vi "InstrumentStudio Plug-In Template.vi"() -> ()   [LabVIEW 2021, in "InstrumentStudio Plug-In Template.lvlib"]
uses:
  InstrumentStudio Plug-In Template.lvlib
  <vilib>/Plug-In SDKs/InstrumentStudio/Plugin Events Enum.ctl
  <vilib>/Plug-In SDKs/InstrumentStudio/Plugin Session.lvclass
  <vilib>/Plug-In SDKs/InstrumentStudio/InstrumentStudio Plugin SDK.lvlib
panel:
  in  "Tab Control":T1(tab)
  in  "Read Selected Sites":bool
  in  "Read Active Pin Map Path":bool
  out "Sites":i32[](array[numeric])
  out "Project Path":path
  in  "Run Write":string
  in  "Write Run Time Config":bool
  in  "Edit Write":string
  in  "Write Edit Time Config":bool
  out "Run Read":string
  in  "Read Run Time Config":bool
  out "Edit Read":string
  in  "Read Edit Time Config":bool
  in  "Read Project Path":bool
  in  "Running":bool
  out "Active Pin Map Path":path
  out "Event Record":i32(listbox)
  in  "Session Id":u64
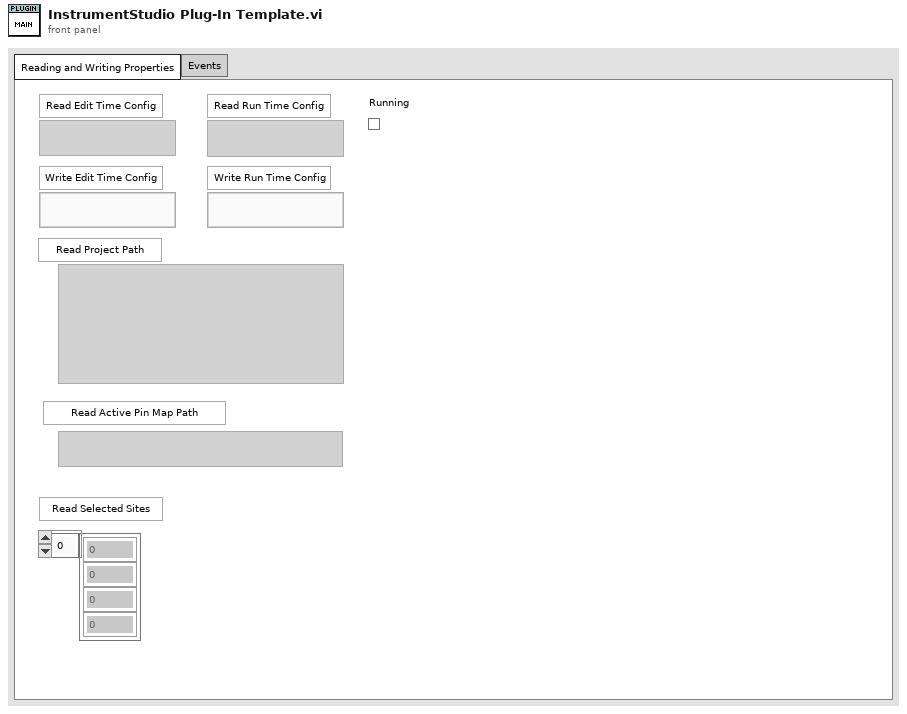
[diagram p1: front panel]
types:
  T1 = enum32{"Reading and Writing Properties", "Events"}
  T2 = typedef "InstrumentStudio Plugin SDK.lvlib/Plugin Events Enum.ctl" = enum32{"Shutdown", "Project Saved", "Stop All Outputs", "Generic Message", "Active Pin Map Changed", "Selected Sites Changed"}
  T3 = typedef "InstrumentStudio Plugin SDK.lvlib/Event Registration Refnum.ctl" = refnum<event-registration>
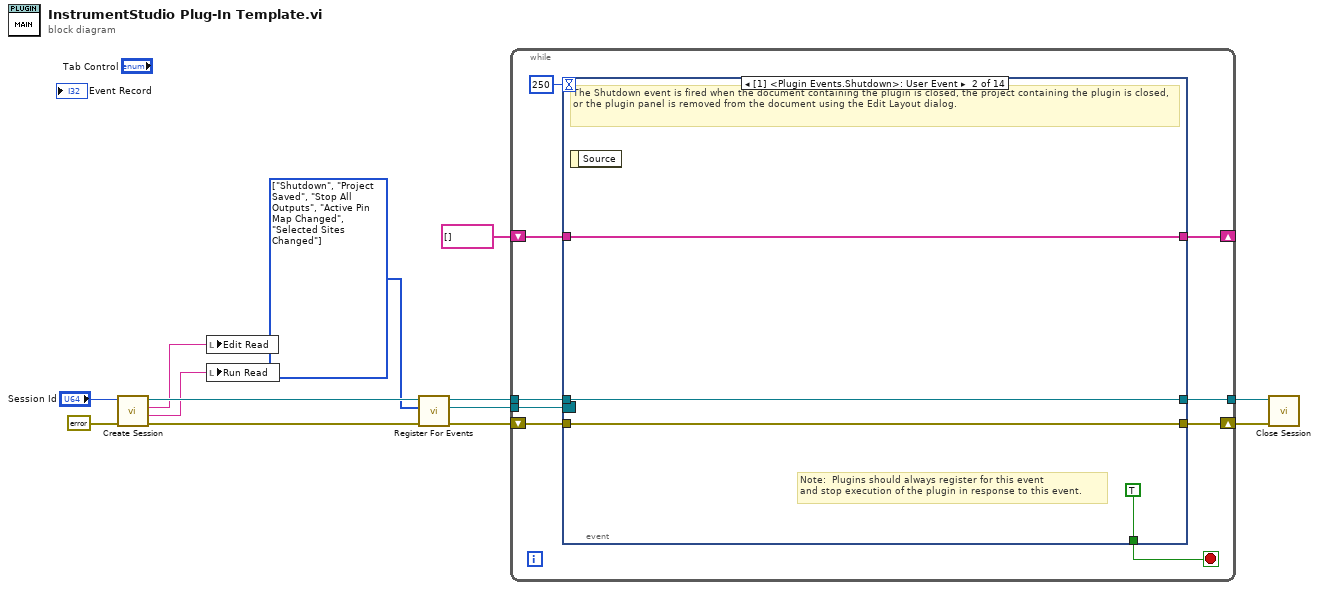
[diagram p0: block diagram]
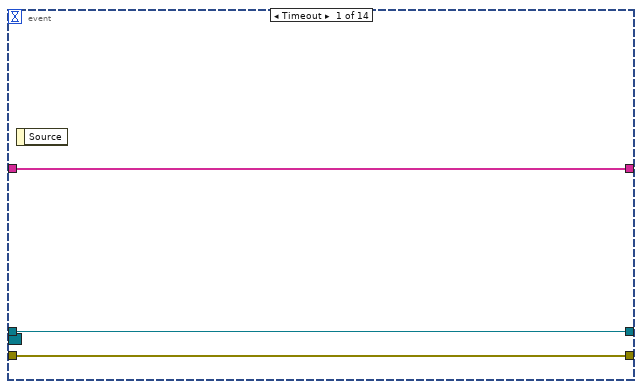
[diagram p2: hidden frame]
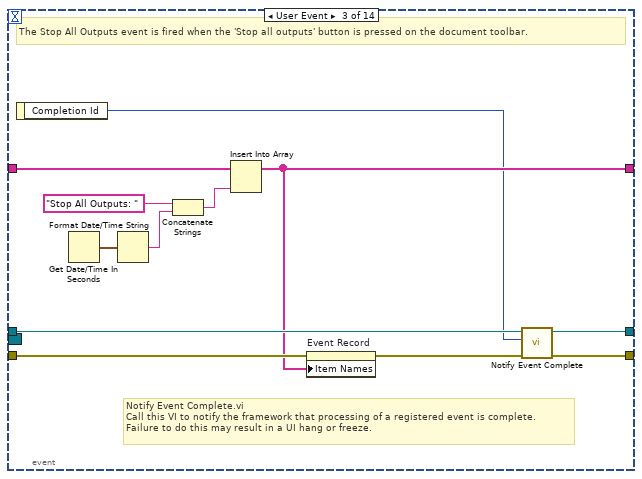
[diagram p3: hidden frame]
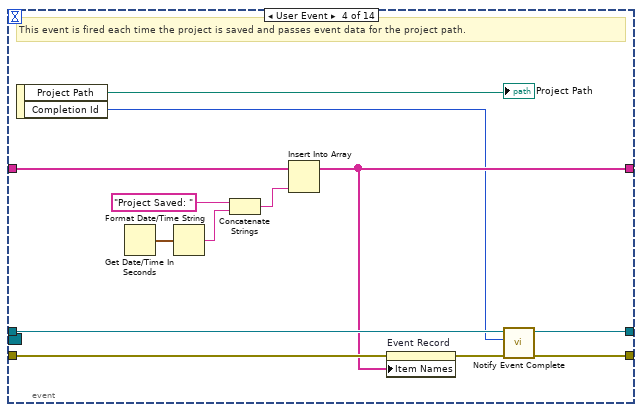
[diagram p4: hidden frame]
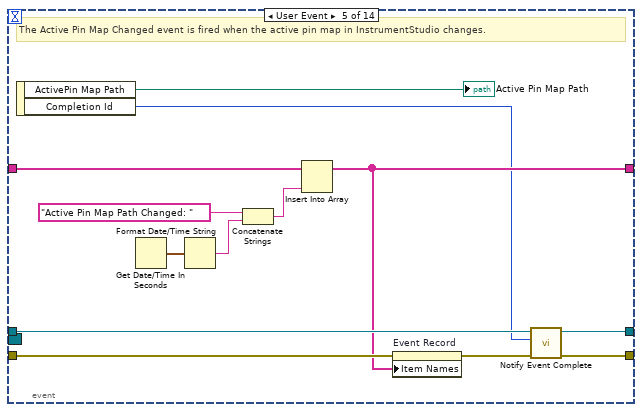
[diagram p5: hidden frame]
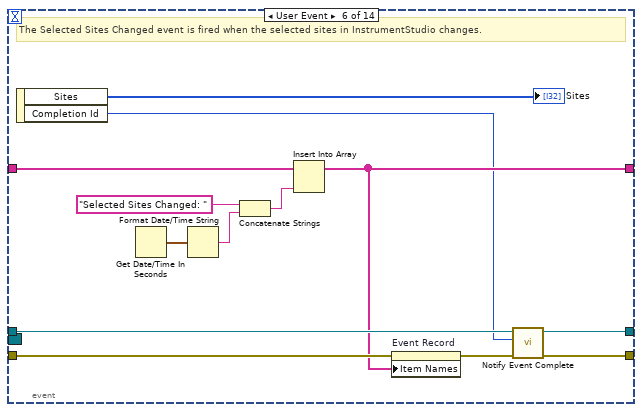
[diagram p6: hidden frame]
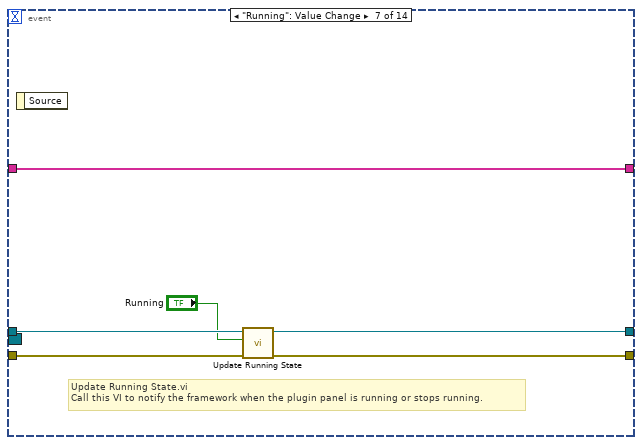
[diagram p7: hidden frame]
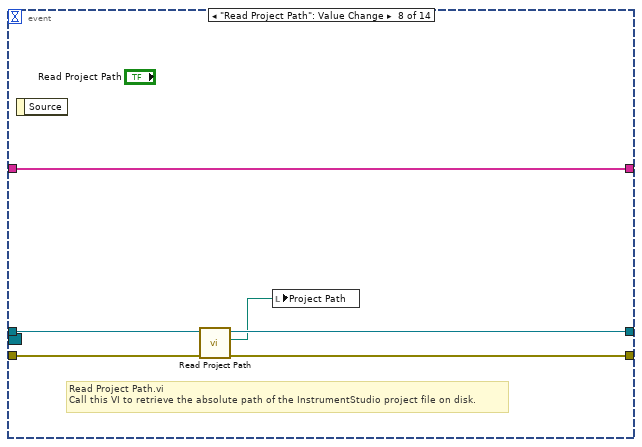
[diagram p8: hidden frame]
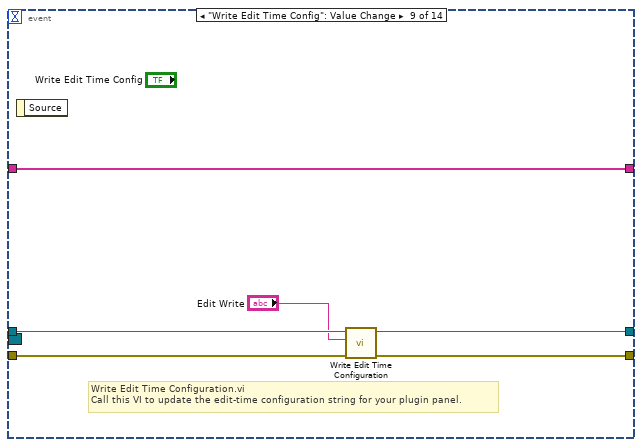
[diagram p9: hidden frame]
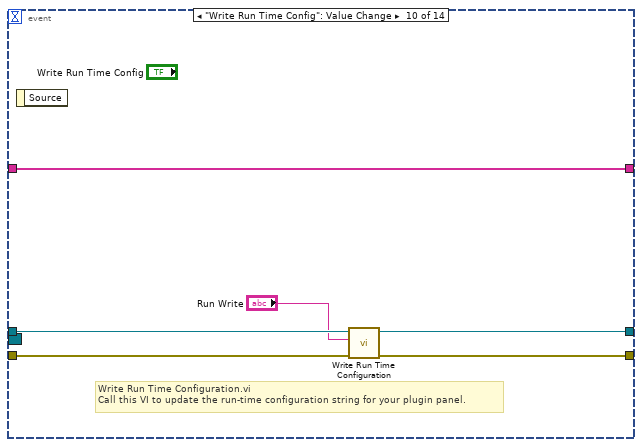
[diagram p10: hidden frame]
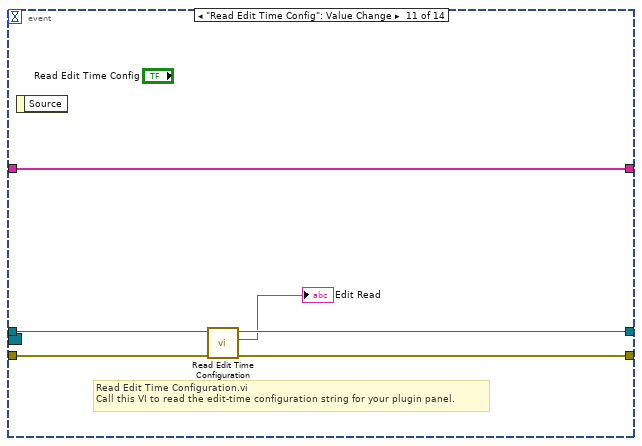
[diagram p11: hidden frame]
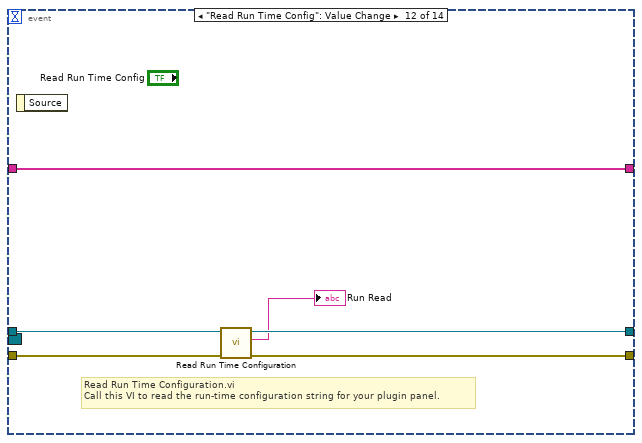
[diagram p12: hidden frame]
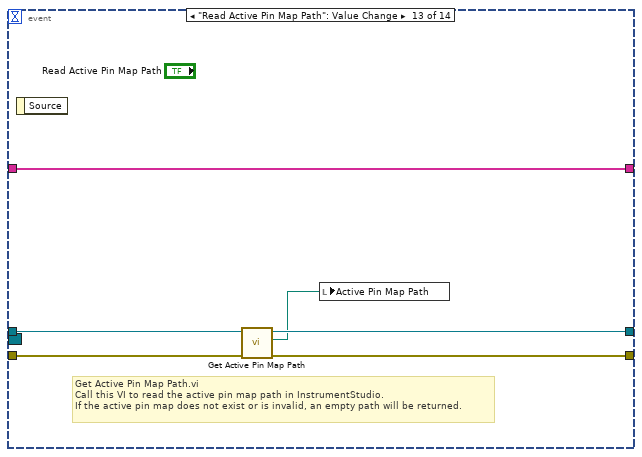
[diagram p13: hidden frame]
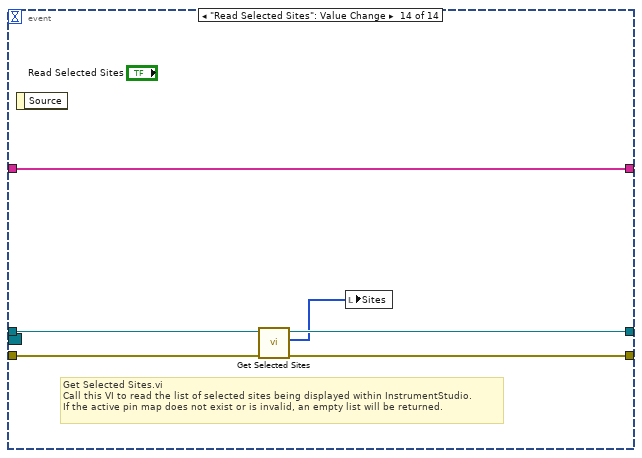
[diagram p14: hidden frame]
diagram:
  w3 = T2[] [enum."Shutdown", enum."Project Saved", enum."Stop All Outputs", enum."Active Pin Map Changed", enum."Selected Sites Changed"] items=["Shutdown", "Project Saved", "Stop All Outputs", "Generic Message", "Active Pin Map Changed", "Selected Sites Changed"] ("Events To Register")
  n1 = call <vilib>:"Create Session.vi"("error in (no error)"=errorcluster {"status"=FALSE, "code"=0, "source"=""}, "Session Id"="Session Id") -> ("error out"=w10:errorcluster, "Run Time Configuration"=w6:string, "Edit Time Configuration"=w5:string, "Session out"=w12:refnum<class "Plugin Session.lvclass">)  [unwired: 5 in, 1 out]
  n2 = local write "Edit Read"(w5) -> ()
  n3 = local write "Run Read"(w6) -> ()
  n4 = call <vilib>:"Register For Events.vi"("error in (no error)"=w10, "Events To Register"=w3, "Session in"=w12) -> ("error out"=w8:errorcluster, "Event Refnum"=w9:T3, "Session out"=w11:refnum<class "Plugin Session.lvclass">)  [unwired: 6 in]
  n5 = while {
    tunnel: w11 -> [w22]
    tunnel: w9 -> [w16]
    shift-right: [w21] -> w1
    shift-left: w8 -> [w18]
    shift-right: [w20] -> _
    shift-left: string[] [] -> [w19]
    tunnel: [w15] -> w2
    stop <- w17 stop-if-true
    n6 = event shown="[1] <Plugin Events.Shutdown>: User Event" {
      selector: w16 -> [_ _ _ _ _ _ _ _ _ _ _ _ _ _]
      dyn-events: _ -> [_ _ _ _ _ _ _ _ _ _ _ _ _ _]
      timeout: 250 -> [_ _ _ _ _ _ _ _ _ _ _ _ _ _]
      tunnel: w22 -> [w25 w29 w41 w54 w67 w79 w86 w92 w97 w100 w106 w112 w121 w127]
      tunnel: [w25 w29 w40 w53 w66 w80 w85 w91 w96 w101 w107 w113 w120 w125] -> w15
      tunnel: [w24 w28 w37 w51 w65 w76 w83 w88 w95 w102 w108 w114 w119 w124] -> w21
      tunnel: [w23 w27 w34 w43 w60 w69 w82 w90 w98 w104 w110 w116 w122 w128] -> w20
      tunnel: w19 -> [w23 w27 w36 w48 w62 w74 w82 w90 w98 w104 w110 w116 w122 w128]
      tunnel: w18 -> [w24 w28 w38 w49 w63 w75 w84 w89 w94 w103 w109 w115 w118 w126]
      tunnel: [_ TRUE _ _ _ _ _ _ _ _ _ _ _ _] -> w17
      event Timeout {
        n7 = event-data() -> ()  [unwired: 1 in, 1 out]
      }
      event User Event {
        # "Note:  Plugins should always register for this event\nand stop execution of the plugin in response to this event."
        # "The Shutdown event is fired when the document containing the plugin is closed, the project containing the plugin is closed, or the plugin panel is removed from the document using the Edit Layout dialog."
        n8 = event-data() -> ()  [unwired: 1 in, 1 out]
      }
      event User Event {
        # "Notify Event Complete.vi\nCall this VI to notify the framework that processing of a registered event is complete. \nFailure to do this may result in a UI hang or freeze."
        # "The Stop All Outputs event is fired when the 'Stop all outputs' button is pressed on the document toolbar."
        n9 = event-data() -> ("Completion Id"=w30:i64)  [unwired: 1 in]
        n10 = Get Date/Time In Seconds() -> (seconds since 1Jan1904=w33:timestamp)
        n11 = Format Date/Time String(seconds (now)=w33) -> (date/time string=w32:string)  [unwired: 2 in]
        n12 = Concatenate Strings("Stop All Outputs: ", w32) -> (w35:string)
        n13 = Insert Into Array(array=w36, new element=w35) -> (w34:string[])  [unwired: 1 in]
        n14 = property on="Event Record" class="LstBox (strict)"(error in=w38, "Item Names"=w34) -> (error out=w39:errorcluster)  [unwired: 1 in, 1 out]
        n15 = call <vilib>:"Notify Event Complete.vi"("error in (no error)"=w39, "Completion Id"=w30, "Session in"=w41) -> ("error out"=w37:errorcluster, "Session out"=w40:refnum<class "Plugin Session.lvclass">)  [unwired: 7 in]
      }
      event User Event {
        # "This event is fired each time the project is saved and passes event data for the project path."
        n16 = event-data() -> ("Project Path"=→"Project Path":path, "Completion Id"=w42:i64)  [unwired: 1 in]
        n17 = Get Date/Time In Seconds() -> (seconds since 1Jan1904=w47:timestamp)
        n18 = Format Date/Time String(seconds (now)=w47) -> (date/time string=w46:string)  [unwired: 2 in]
        n19 = Concatenate Strings("Project Saved: ", w46) -> (w44:string)
        n20 = Insert Into Array(array=w48, new element=w44) -> (w43:string[])  [unwired: 1 in]
        n21 = property on="Event Record" class="LstBox (strict)"(error in=w49, "Item Names"=w43) -> (error out=w50:errorcluster)  [unwired: 1 in, 1 out]
        n22 = call <vilib>:"Notify Event Complete.vi"("error in (no error)"=w50, "Completion Id"=w42, "Session in"=w54) -> ("error out"=w51:errorcluster, "Session out"=w53:refnum<class "Plugin Session.lvclass">)  [unwired: 7 in]
      }
      event User Event {
        # "The Active Pin Map Changed event is fired when the active pin map in InstrumentStudio changes."
        n23 = event-data() -> ("ActivePin Map Path"=→"Active Pin Map Path":path, "Completion Id"=w55:i64)  [unwired: 1 in]
        n24 = Get Date/Time In Seconds() -> (seconds since 1Jan1904=w59:timestamp)
        n25 = Format Date/Time String(seconds (now)=w59) -> (date/time string=w57:string)  [unwired: 2 in]
        n26 = Concatenate Strings("Active Pin Map Path Changed: ", w57) -> (w56:string)
        n27 = Insert Into Array(array=w62, new element=w56) -> (w60:string[])  [unwired: 1 in]
        n28 = property on="Event Record" class="LstBox (strict)"(error in=w63, "Item Names"=w60) -> (error out=w64:errorcluster)  [unwired: 1 in, 1 out]
        n29 = call <vilib>:"Notify Event Complete.vi"("error in (no error)"=w64, "Completion Id"=w55, "Session in"=w67) -> ("error out"=w65:errorcluster, "Session out"=w66:refnum<class "Plugin Session.lvclass">)  [unwired: 7 in]
      }
      event User Event {
        # "The Selected Sites Changed event is fired when the selected sites in InstrumentStudio changes."
        n30 = event-data() -> ("Sites"=→"Sites":i32[], "Completion Id"=w68:i64)  [unwired: 1 in]
        n31 = Get Date/Time In Seconds() -> (seconds since 1Jan1904=w71:timestamp)
        n32 = Format Date/Time String(seconds (now)=w71) -> (date/time string=w72:string)  [unwired: 2 in]
        n33 = Concatenate Strings("Selected Sites Changed: ", w72) -> (w73:string)
        n34 = Insert Into Array(array=w74, new element=w73) -> (w69:string[])  [unwired: 1 in]
        n35 = property on="Event Record" class="LstBox (strict)"(error in=w75, "Item Names"=w69) -> (error out=w77:errorcluster)  [unwired: 1 in, 1 out]
        n36 = call <vilib>:"Notify Event Complete.vi"("error in (no error)"=w77, "Completion Id"=w68, "Session in"=w79) -> ("error out"=w76:errorcluster, "Session out"=w80:refnum<class "Plugin Session.lvclass">)  [unwired: 7 in]
      }
      event "Running": Value Change {
        # "Update Running State.vi\nCall this VI to notify the framework when the plugin panel is running or stops running."
        n37 = event-data() -> ()  [unwired: 1 in, 1 out]
        n38 = call <vilib>:"Update Running State.vi"("error in (no error)"=w84, "Is Running"="Running", "Plugin Session in"=w86) -> ("error out"=w83:errorcluster, "Plugin Session out"=w85:refnum<class "Plugin Session.lvclass">)  [unwired: 7 in]
      }
      event "Read Project Path": Value Change {
        # "Read Project Path.vi\nCall this VI to retrieve the absolute path of the InstrumentStudio project file on disk."
        n39 = event-data() -> ()  [unwired: 1 in, 1 out]
        n40 = call <vilib>:"Read Project Path.vi"("error in (no error)"=w89, "Session in"=w92) -> ("error out"=w88:errorcluster, "Project Path"=w87:path, "Session out"=w91:refnum<class "Plugin Session.lvclass">)  [unwired: 7 in]
        n41 = local write "Project Path"(w87) -> ()
      }
      event "Write Edit Time Config": Value Change {
        # "Write Edit Time Configuration.vi\nCall this VI to update the edit-time configuration string for your plugin panel."
        n42 = event-data() -> ()  [unwired: 1 in, 1 out]
        n43 = call <vilib>:"Write Edit Time Configuration.vi"("error in (no error)"=w94, "Edit Time Configuration"="Edit Write", "Session in"=w97) -> ("error out"=w95:errorcluster, "Session out"=w96:refnum<class "Plugin Session.lvclass">)  [unwired: 7 in]
      }
      event "Write Run Time Config": Value Change {
        # "Write Run Time Configuration.vi\nCall this VI to update the run-time configuration string for your plugin panel."
        n44 = event-data() -> ()  [unwired: 1 in, 1 out]
        n45 = call <vilib>:"Write Run Time Configuration.vi"("error in (no error)"=w103, "Run Time Configuration"="Run Write", "Session in"=w100) -> ("error out"=w102:errorcluster, "Session out"=w101:refnum<class "Plugin Session.lvclass">)  [unwired: 7 in]
      }
      event "Read Edit Time Config": Value Change {
        # "Read Edit Time Configuration.vi\nCall this VI to read the edit-time configuration string for your plugin panel."
        n46 = event-data() -> ()  [unwired: 1 in, 1 out]
        n47 = call <vilib>:"Read Edit Time Configuration.vi"("error in (no error)"=w109, "Session in"=w106) -> ("error out"=w108:errorcluster, "Edit Time Configuration"=→"Edit Read":string, "Session out"=w107:refnum<class "Plugin Session.lvclass">)  [unwired: 7 in]
      }
      event "Read Run Time Config": Value Change {
        # "Read Run Time Configuration.vi\nCall this VI to read the run-time configuration string for your plugin panel."
        n48 = event-data() -> ()  [unwired: 1 in, 1 out]
        n49 = call <vilib>:"Read Run Time Configuration.vi"("error in (no error)"=w115, "Session in"=w112) -> ("error out"=w114:errorcluster, "Run Time Configuration"=→"Run Read":string, "Session out"=w113:refnum<class "Plugin Session.lvclass">)  [unwired: 7 in]
      }
      event "Read Active Pin Map Path": Value Change {
        # "Get Active Pin Map Path.vi\nCall this VI to read the active pin map path in InstrumentStudio. \nIf the active pin map does not exist or is invalid, an empty path will be returned."
        n50 = event-data() -> ()  [unwired: 1 in, 1 out]
        n51 = call-dynamic "Get Active Pin Map Path.vi"("error in (no error)"=w118, "Session in"=w121) -> ("error out"=w119:errorcluster, "Active Pin Map Path"=w117:path, "Session out"=w120:refnum<class "Plugin Session.lvclass">)  [unwired: 7 in]
        n52 = local write "Active Pin Map Path"(w117) -> ()
      }
      event "Read Selected Sites": Value Change {
        # "Get Selected Sites.vi\nCall this VI to read the list of selected sites being displayed within InstrumentStudio.\nIf the active pin map does not exist or is invalid, an empty list will be returned."
        n53 = event-data() -> ()  [unwired: 1 in, 1 out]
        n54 = call-dynamic "Get Selected Sites.vi"("error in (no error)"=w126, "Session in"=w127) -> ("error out"=w124:errorcluster, "Selected Sites"=w123:i32[], "Session out"=w125:refnum<class "Plugin Session.lvclass">)  [unwired: 7 in]
        n55 = local write "Sites"(w123) -> ()
      }
    }
  }
  n56 = call <vilib>:"Close Session.vi"("error in (no error)"=w1, "Session in"=w2) -> ()  [unwired: 9 in, 1 out]
